vi "All SubFunctions 5.vi"(8 "error":errorcluster, 9 "lines 1":tag="PXI1Slot8/port0/line2", 10 "lines":tag="PXI1Slot8/port0/line3", 11 "Path for Log":path) -> (0 "error IO":errorcluster, 1 "appended array 1":string[][](array[string]), 2 "appended array":string[][](array[string]))   [LabVIEW 2014]
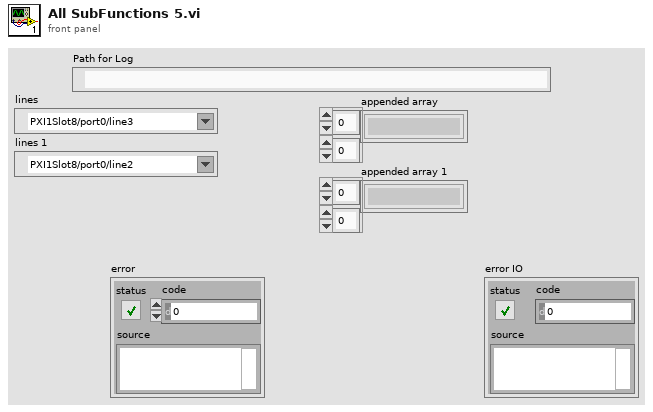
[diagram p1: front panel]
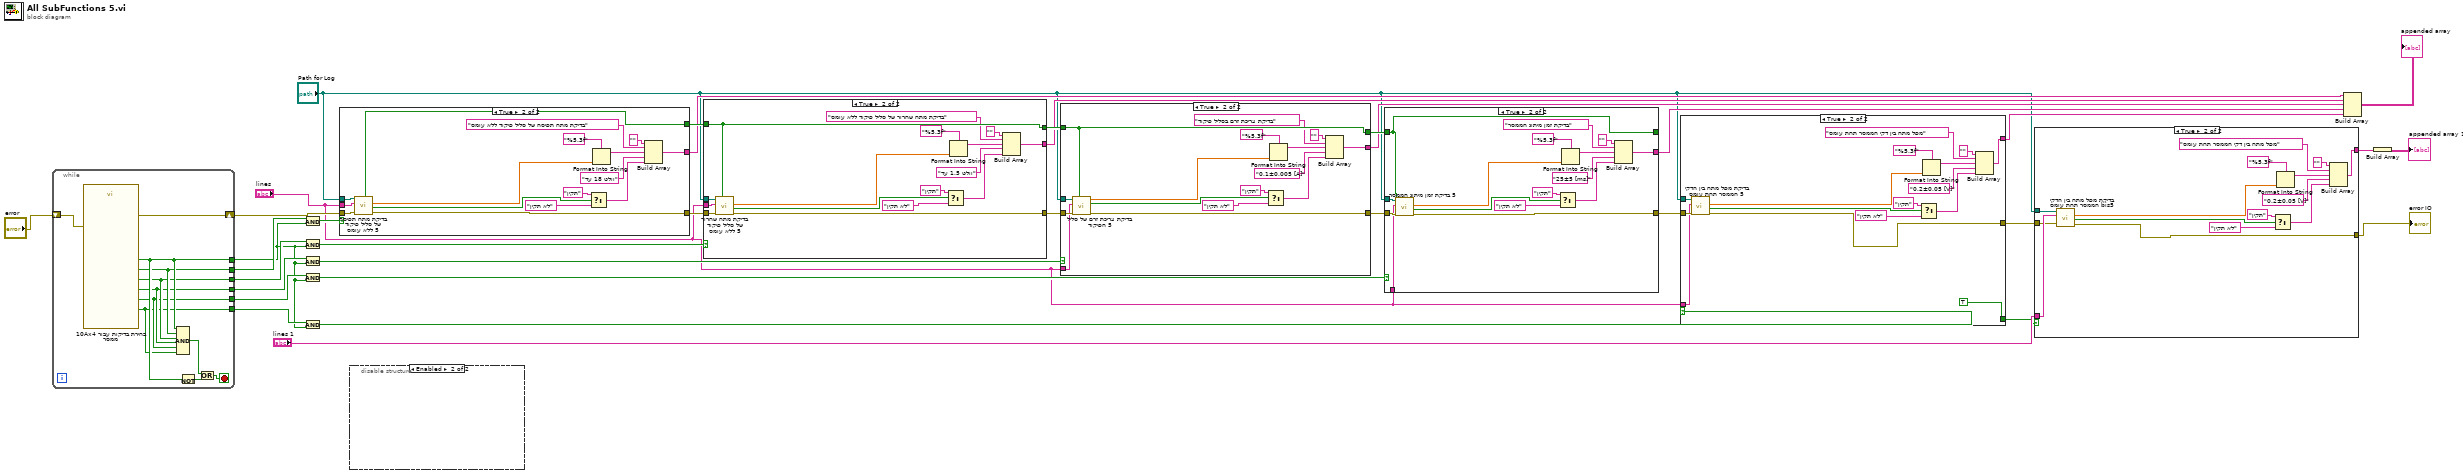
[diagram p0: block diagram]
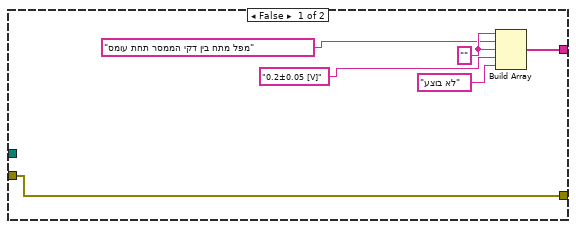
[diagram p2: hidden frame]
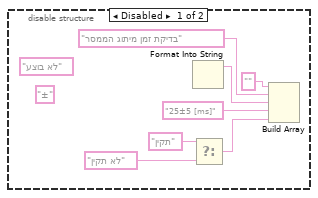
[diagram p3: hidden frame]
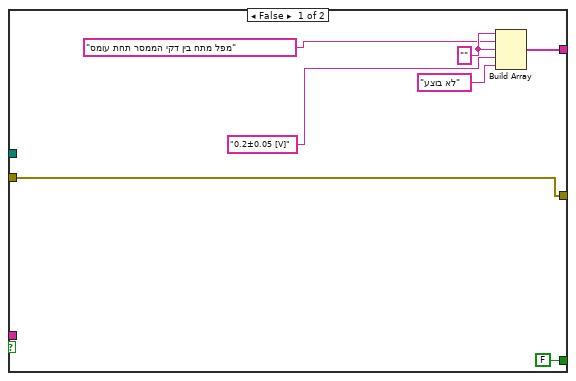
[diagram p4: hidden frame]
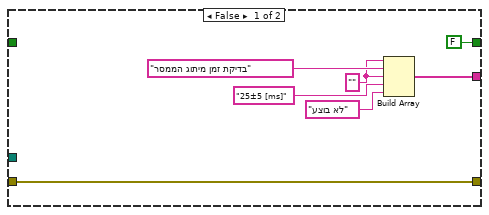
[diagram p5: hidden frame]
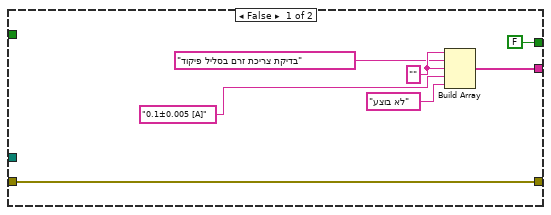
[diagram p6: hidden frame]
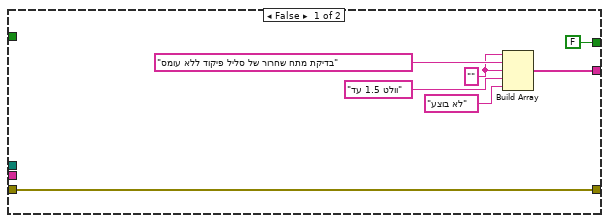
[diagram p7: hidden frame]
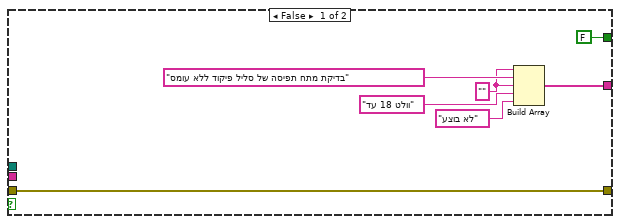
[diagram p8: hidden frame]
diagram:
  n1 = while {
    tunnel: [w38] -> w28
    tunnel: [w37] -> w26
    tunnel: [w36] -> w24
    tunnel: [w35] -> w22
    tunnel: [w39] -> w21
    tunnel: [w40] -> w20
    shift-right: [w44] -> w30
    shift-left: "error" -> [w45]
    stop <- w43 stop-if-true
    n2 = call "10Ax4 בחירת בדיקות עבור ממסר.vi"("error in (no error)"=w45) -> ("בדיקת מפל מתח בין דקי הממסר תחת עומס"=w35:bool, "בדיקת זמן מיתוג הממסר"=w36:bool, "בדיקת צריכת זרם של סליל הפיקוד"=w37:bool, "בדיקת מתח שחרור של סליל פיקוד ללא עומס"=w38:bool, "בדיקת מתח תפיסה של סליל פיקוד ללא עומס"=w39:bool, "OK"=w40:bool, "error out"=w44:errorcluster)  [unwired: 11 in, 1 out]
    n3 = Compound Arithmetic op=AND(w40, w39, w38, w37, w36, w35) -> (w41:bool)
    n4 = Not(x=w40) -> (.not. x?=w42:bool)
    n5 = Or(x=w41, y=w42) -> (x .or. y?=w43:bool)
  }
  n6 = And(x=w21, y=w20) -> (x .and. y?=w29:bool)
  n7 = And(x=w28, y=w20) -> (x .and. y?=w27:bool)
  n8 = And(x=w26, y=w20) -> (x .and. y?=w25:bool)
  n9 = And(x=w24, y=w20) -> (x .and. y?=w23:bool)
  n10 = And(x=w22, y=w20) -> (x .and. y?=w7:bool)
  n11 = case shown="True" w29 {
    tunnel: [w52 w68] -> w32
    tunnel: w30 -> [w52 w67]
    tunnel: "Path for Log" -> [_ w66]
    tunnel: [FALSE ("resultUserPrompt") w65] -> w19
    tunnel: [w48 w55] -> w16
    tunnel: "lines" -> [_ w53]
    frame False {
      w47 = "" ("element")
      n12 = Build Array(w47, "בדיקת מתח תפיסה של סליל פיקוד ללא עומס" ("element"), w47, "עד 18 וולט" ("element"), "לא בוצע") -> (w48:string[])
    }
    frame True {
      n13 = call "בדיקת מתח תפיסה של סליל פיקוד ללא עומס 5.vi"("error"=w67, "lines"=w53, "Path for Log"=w66) -> ("error out"=w68:errorcluster, "מצב ממסר פתוח/סגור"=w62:bool, "מתח סגירת הממסר"=w61:dbl, "resultUserPrompt"=w65:bool)  [unwired: 4 in, 1 out]
      n14 = Select(t="תקין", s=w62, f="לא תקין") -> (s? t:f=w56:string)
      n15 = Format Into String(format string="%5.3f", w61) -> (resulting string=w57:string)  [unwired: 2 in, 1 out]
      n16 = Build Array("" ("element"), "בדיקת מתח תפיסה של סליל פיקוד ללא עומס" ("element"), w57, "עד 18 וולט" ("element"), w56) -> (w55:string[])
    }
  }
  n17 = disable-structure shown="Enabled" {
    frame Disabled {
      (unwired) "±"
      (unwired) "לא בוצע"
      n18 = Format Into String() -> (resulting string=w73:string)  [unwired: 4 in, 1 out]
      n19 = Select(t="תקין", f="לא תקין") -> (s? t:f=w75:string)  [unwired: 1 in]
      n20 = Build Array("" ("element"), "בדיקת זמן מיתוג הממסר" ("element"), w73, "25±5 [ms]" ("element"), w75) -> ()  [unwired: 1 out]
    }
    frame Enabled {
    }
  }
  n21 = case shown="True" w27 {
    tunnel: w32 -> [w82 w98]
    tunnel: [w82 w97] -> w31
    tunnel: "Path for Log" -> [_ w96]
    tunnel: w19 -> [_ w95]
    tunnel: [FALSE ("resultUserPrompt") w95] -> w18
    tunnel: [w76 w85] -> w15
    tunnel: "lines" -> [_ w83]
    frame False {
      w77 = "" ("element")
      n22 = Build Array(w77, "בדיקת מתח שחרור של סליל פיקוד ללא עומס" ("element"), w77, "עד 1.5 וולט" ("element"), "לא בוצע") -> (w76:string[])
    }
    frame True {
      n23 = call "בדיקת מתח שחרור של סליל פיקוד ללא עומס 5.vi"("userResult"=w95, "error"=w98, "lines"=w83, "Path for Log"=w96) -> ("error out"=w97:errorcluster, "מצב ממסר פתוח/סגור"=w91:bool, "מתח פתיחת הממסר"=w92:dbl)  [unwired: 4 in, 1 out]
      n24 = Select(t="תקין", s=w91, f="לא תקין") -> (s? t:f=w86:string)
      n25 = Format Into String(format string="%5.3f", w92) -> (resulting string=w88:string)  [unwired: 2 in, 1 out]
      n26 = Build Array("" ("element"), "בדיקת מתח שחרור של סליל פיקוד ללא עומס" ("element"), w88, "עד 1.5 וולט" ("element"), w86) -> (w85:string[])
    }
  }
  n27 = case shown="True" w25 {
    tunnel: [w105 w121] -> w33
    tunnel: w31 -> [w105 w120]
    tunnel: "Path for Log" -> [_ w119]
    tunnel: w18 -> [_ w118]
    tunnel: [FALSE ("resultUserPrompt") w118] -> w17
    tunnel: [w100 w108] -> w14
    tunnel: "lines" -> [_ w106]
    frame False {
      w103 = "" ("element")
      n28 = Build Array(w103, "בדיקת צריכת זרם בסליל פיקוד" ("element"), w103, "0.1±0.005 [A]" ("element"), "לא בוצע") -> (w100:string[])
    }
    frame True {
      n29 = call "בדיקת צריכת זרם של סליל הפיקוד 5.vi"("resultUserPrompt"=w118, "error"=w120, "lines"=w106, "Path for Log"=w119) -> ("error out"=w121:errorcluster, "צריכת זרם בסליל בטווח כן/לא"=w111:bool, "צריכת זרם בסליל"=w112:dbl)  [unwired: 5 in]
      n30 = Select(t="תקין", s=w111, f="לא תקין") -> (s? t:f=w110:string)
      n31 = Format Into String(format string="%5.3f", w112) -> (resulting string=w109:string)  [unwired: 2 in, 1 out]
      n32 = Build Array("" ("element"), "בדיקת צריכת זרם בסליל פיקוד" ("element"), w109, "0.1±0.005 [A]" ("element"), w110) -> (w108:string[])
    }
  }
  n33 = case shown="True" w23 {
    tunnel: w33 -> [w128 w144]
    tunnel: [w128 w143] -> w12
    tunnel: "Path for Log" -> [_ w142]
    tunnel: w17 -> [_ w130]
    tunnel: [FALSE ("resultUserPrompt") w130] -> _
    tunnel: [w122 w132] -> w13
    tunnel: "lines" -> [_ w129]
    frame False {
      w124 = "" ("element")
      n34 = Build Array(w124, "בדיקת זמן מיתוג הממסר" ("element"), w124, "25±5 [ms]" ("element"), "לא בוצע") -> (w122:string[])
    }
    frame True {
      n35 = call "בדיקת זמן מיתוג הממסר 5.vi"("resultUserPrompt"=w130, "error"=w144, "lines"=w129, "Path for Log"=w142) -> ("error out"=w143:errorcluster, "בטוח כן/לא"=w134:bool, "בדיקת זמן מיתוג הממסר"=w133:dbl)  [unwired: 5 in]
      n36 = Select(t="תקין", s=w134, f="לא תקין") -> (s? t:f=w135:string)
      n37 = Format Into String(format string="%5.3f", w133) -> (resulting string=w137:string)  [unwired: 2 in, 1 out]
      n38 = Build Array("" ("element"), "בדיקת זמן מיתוג הממסר" ("element"), w137, "25±5 [ms]" ("element"), w135) -> (w132:string[])
    }
  }
  n39 = case shown="True" w7 {
    tunnel: [w151 w152] -> w6
    tunnel: w12 -> [w151 w167]
    tunnel: "Path for Log" -> [_ w166]
    tunnel: [w148 w156] -> w11
    tunnel: "lines" -> [_ w154]
    tunnel: [FALSE TRUE] -> w2
    frame False {
      w149 = "" ("element")
      n40 = Build Array(w149, "מפל מתח בין דקי הממסר תחת עומס" ("element"), w149, "0.2±0.05 [V]" ("element"), "לא בוצע") -> (w148:string[])
    }
    frame True {
      n41 = call "בדיקת מפל מתח בין הדקי הממסר תחת עומס 5.vi"("error"=w167, "lines"=w154, "Path for Log"=w166) -> ("error IO"=w152:errorcluster, "בטוח כן/לא"=w157:bool, "מפל מתח בין דקי הממסר תחת עומס"=w158:dbl)  [unwired: 5 in, 1 out]
      n42 = Select(t="תקין", s=w157, f="לא תקין") -> (s? t:f=w159:string)
      n43 = Format Into String(format string="%5.3f", w158) -> (resulting string=w161:string)  [unwired: 2 in, 1 out]
      n44 = Build Array("" ("element"), "מפל מתח בין דקי הממסר תחת עומס" ("element"), w161, "0.2±0.05 [V]" ("element"), w159) -> (w156:string[])
    }
  }
  n45 = case shown="True" w2 {
    tunnel: [w170 w174] -> w5
    tunnel: "Path for Log" -> [_ w188]
    tunnel: [w171 w178] -> w4
    tunnel: "lines 1" -> [_ w176]
    tunnel: w6 -> [w170 w175]
    frame False {
      w172 = "" ("element")
      n46 = Build Array(w172, "מפל מתח בין דקי הממסר תחת עומס" ("element"), w172, "0.2±0.05 [V]" ("element"), "לא בוצע") -> (w171:string[])
    }
    frame True {
      n47 = call "בדיקת מפל מתח בין הדקי הממסר תחת עומס bis5.vi"("error"=w175, "lines"=w176, "Path for Log"=w188) -> ("error IO"=w174:errorcluster, "בטוח כן/לא"=w179:bool, "מפל מתח בין דקי הממסר תחת עומס"=w180:dbl)  [unwired: 5 in, 1 out]
      n48 = Select(t="תקין", s=w179, f="לא תקין") -> (s? t:f=w181:string)
      n49 = Format Into String(format string="%5.3f", w180) -> (resulting string=w183:string)  [unwired: 2 in, 1 out]
      n50 = Build Array("" ("element"), "מפל מתח בין דקי הממסר תחת עומס" ("element"), w183, "0.2±0.05 [V]" ("element"), w181) -> (w178:string[])
    }
  }
  "error IO" <- w5
  n51 = Build Array(w16, w15, w14, w13, w11) -> (→"appended array":string[][])
  n52 = Build Array(w4) -> (→"appended array 1":string[][])
